vi "xcorr bkp enable.vi"(4 "shift":u8, 5 "Pulse Energy":fxp<+,32,0>=0.99609375, 6 "N":u8, 7 "y":u32, 8 "x":u32, 9 "enable":bool, 10 "lag":u16) -> (1 "Rxy valid":bool, 2 "Rxy":u64, 3 "trigger":bool)   [LabVIEW 2017]
uses:
  <vilib>/rvi/FXPMathLib/basic elements/FxpDiscreteDelay/XNode/nifxpmath_DiscreteDelay.xnode
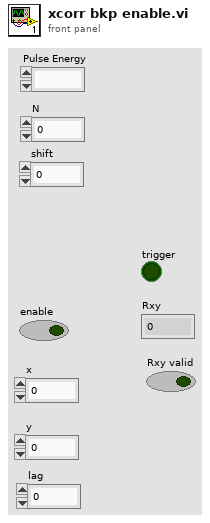
[diagram p1: front panel]
types:
  T1 = cluster{"Q":bool, "Q":bool, "Q":bool, "Q":bool, "Q":bool, "Q":bool, "Q":bool, "Q":bool, "Q":bool, "Q":bool, "Q":bool, "Q":bool, "valid":bool}
  T2 = cluster{"Q":bool, "Q":bool, "Q":bool, "Q":bool, "Q":bool, "Q":bool, "Q":bool, "Q":bool, "Q":bool, "Q":bool, "Q":bool, "Q":bool, "Q":bool}
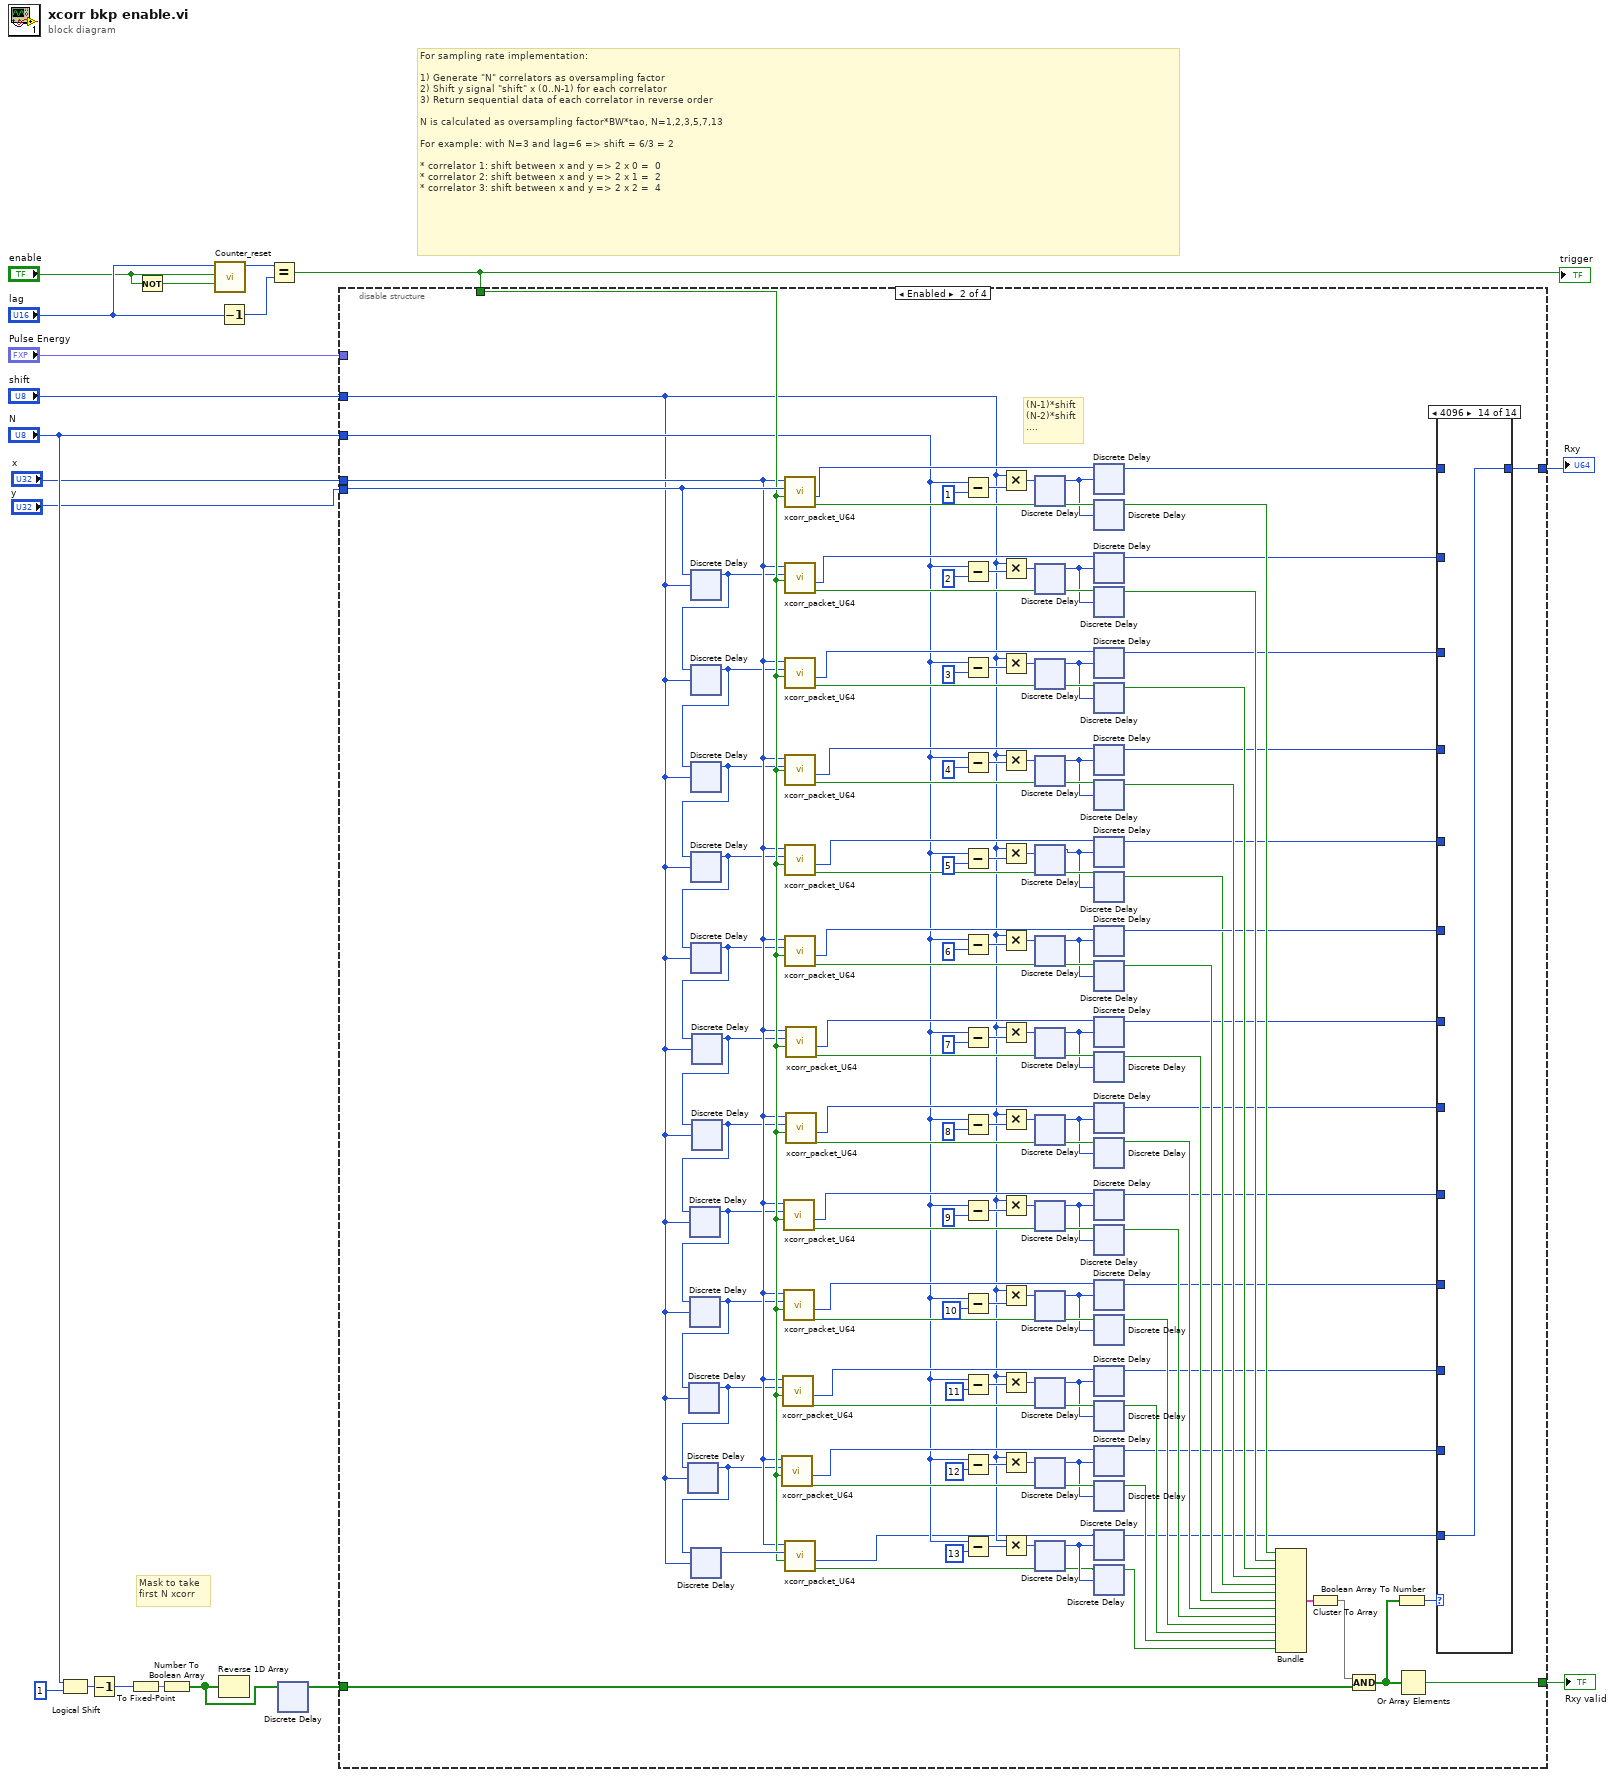
[diagram p0: block diagram]
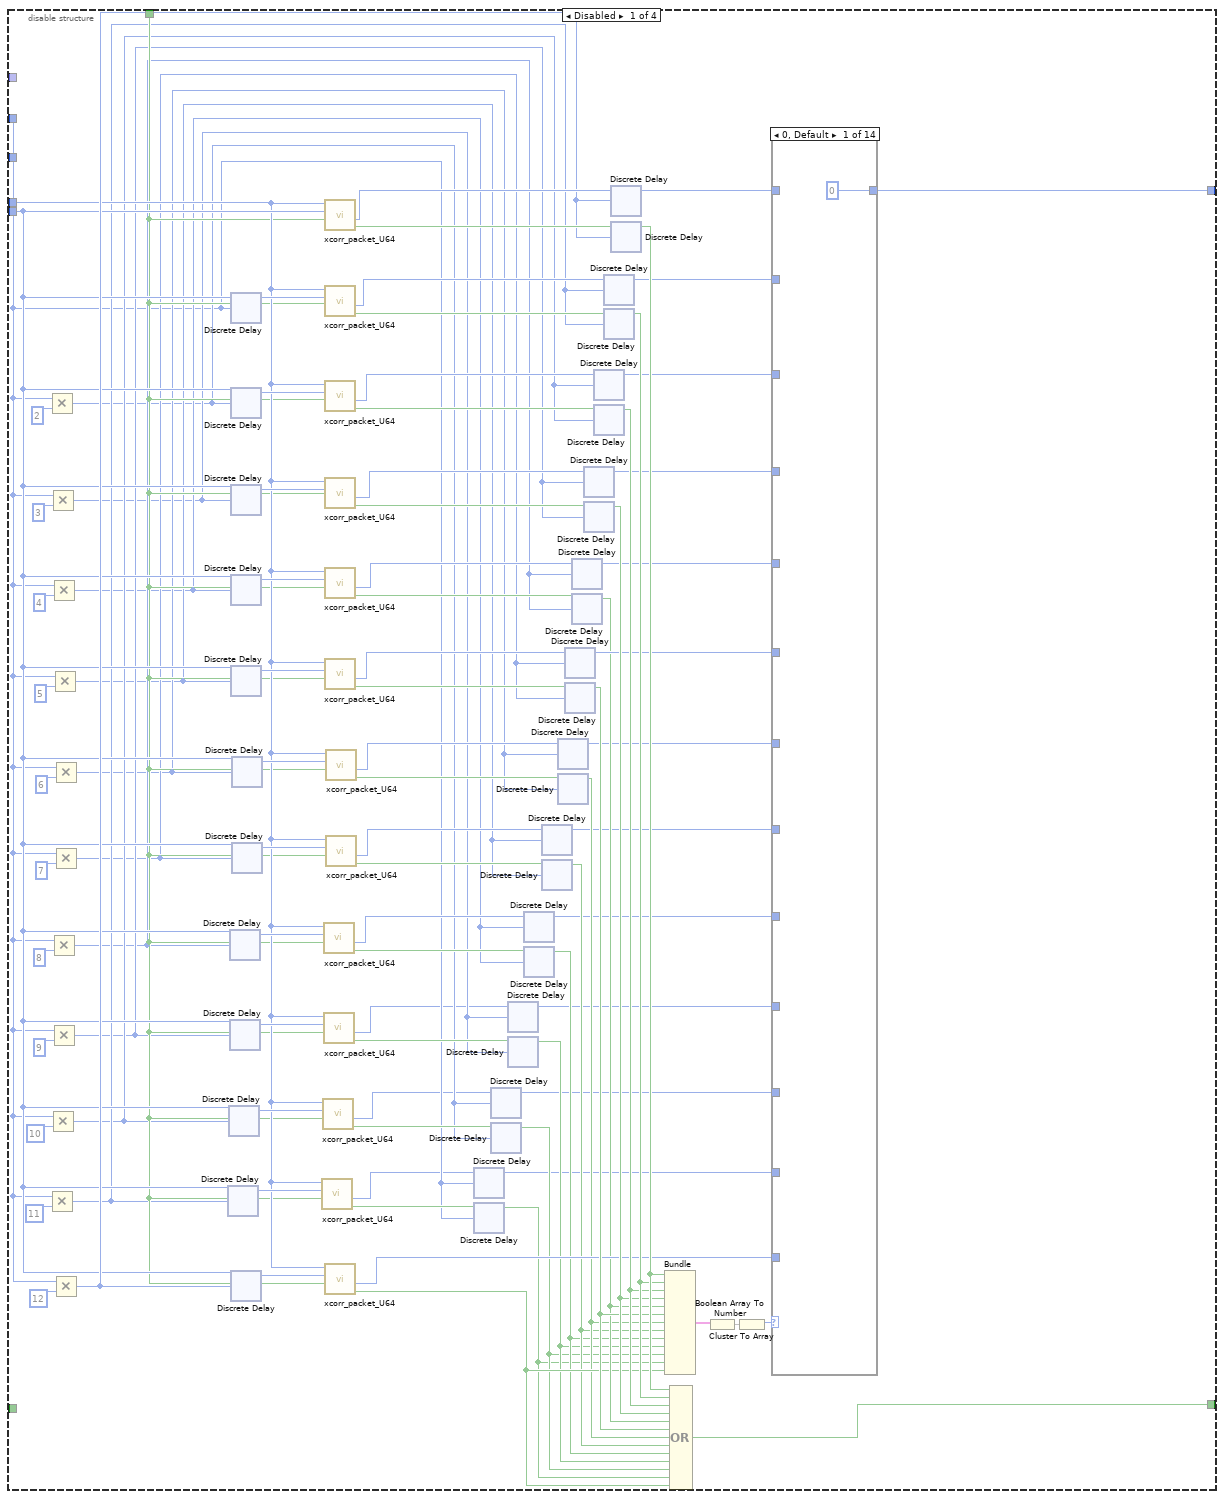
[diagram p2: hidden frame]
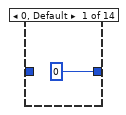
[diagram p16: hidden frame]
diagram:
  # "Mask to take \nfirst N xcorr"
  # "For sampling rate implementation:\n\n1) Generate \"N\" correlators as oversampling factor\n2) Shift y signal \"shift\" x (0..N-1) for each correlator\n3) Return sequential data of each correlator in reverse order\n\nN is calculated as oversampling factor*BW*tao, N=1,2,3,5,7,13\n\nFor example: with N=3 and lag=6 => shift = 6/3 = 2\n\n* correlator 1: shift between x and y => 2 x 0 =  0\n* correlator 2: shift between x and y => 2 x 1 =  2\n* correlator 3: shift between x and y => 2 x 2 =  4"
  n1 = Logical Shift(y="N", x=u16 1) -> (x << y=w8:u16)
  n2 = Decrement(x=w8) -> (x-1=w7:u16)
  n3 = To Fixed-Point(number=w7) -> (fixed-point=w6:fxp<+,13,13>)  [unwired: 1 in]
  n4 = Not(x="enable") -> (.not. x?=w17:bool)
  n5 = Number To Boolean Array(number=w6) -> (Boolean array=w4:bool[])
  n6 = call "Counter_reset.vi"("reset"=w17, "enable"="enable", "limit"="lag") -> ("count"=w18:u16)  [unwired: 8 in]
  n7 = Decrement(x="lag") -> (x-1=w15:u16)
  n8 = Reverse 1D Array(array=w4) -> ()  [unwired: 1 out]
  n9 = Equal?(x=w18, y=w15) -> (x = y?=w12:bool)
  "trigger" <- w12
  n10 = xnode ("Discrete Delay")("D"=w4) -> ("Q"=w10:bool[])
  n11 = disable-structure shown="Enabled" {
    disable-tunnel: [w112 w188 w355 _] -> w19
    disable-tunnel: [w107 w251 w416 _] -> w14
    disable-tunnel: "y" -> [w42 w211 w270 _]
    disable-tunnel: "x" -> [w41 w200 w273 _]
    disable-tunnel: w12 -> [w40 w210 w376 _]
    disable-tunnel: "shift" -> [w28 w131 w298 _]
    disable-tunnel: w10 -> [_ w187 w354 _]
    disable-tunnel: "N" -> [_ w156 w323 _]
    disable-tunnel: "Pulse Energy" -> [_ _ w269 _]
    frame Disabled {
      n12 = Multiply(x=w28, y=u8 2 ("x")) -> (x*y=w29:u8)
      n13 = Multiply(x=w28, y=u8 11 ("x")) -> (x*y=w38:u8)
      n14 = Multiply(x=w28, y=u8 3 ("x")) -> (x*y=w30:u8)
      n15 = Multiply(x=w28, y=u8 10 ("x")) -> (x*y=w37:u8)
      n16 = Multiply(x=w28, y=u8 4 ("x")) -> (x*y=w31:u8)
      n17 = Multiply(x=w28, y=u8 8 ("x")) -> (x*y=w35:u8)
      n18 = Multiply(x=w28, y=u8 9 ("x")) -> (x*y=w36:u8)
      n19 = Multiply(x=w28, y=u8 5 ("x")) -> (x*y=w32:u8)
      n20 = Multiply(x=w28, y=u8 6 ("x")) -> (x*y=w33:u8)
      n21 = Multiply(x=w28, y=u8 7 ("x")) -> (x*y=w34:u8)
      n22 = Multiply(x=w28, y=u8 12 ("x")) -> (x*y=w78:u8)
      n23 = xnode ("Discrete Delay")("D"=w42, "n-1[0..255]"=w38) -> ("Q"=w44:u32)
      n24 = xnode ("Discrete Delay")("D"=w42, "n-1[0..255]"=w37) -> ("Q"=w51:u32)
      n25 = xnode ("Discrete Delay")("D"=w42, "n-1[0..255]"=w35) -> ("Q"=w57:u32)
      n26 = xnode ("Discrete Delay")("D"=w42, "n-1[0..255]"=w36) -> ("Q"=w54:u32)
      n27 = xnode ("Discrete Delay")("D"=w42, "n-1[0..255]"=w28) -> ("Q"=w111:u32)
      n28 = xnode ("Discrete Delay")("D"=w42, "n-1[0..255]"=w29) -> ("Q"=w105:u32)
      n29 = xnode ("Discrete Delay")("D"=w42, "n-1[0..255]"=w30) -> ("Q"=w103:u32)
      n30 = xnode ("Discrete Delay")("D"=w42, "n-1[0..255]"=w31) -> ("Q"=w101:u32)
      n31 = xnode ("Discrete Delay")("D"=w42, "n-1[0..255]"=w32) -> ("Q"=w87:u32)
      n32 = xnode ("Discrete Delay")("D"=w42, "n-1[0..255]"=w78) -> ("Q"=w79:u32)
      n33 = xnode ("Discrete Delay")("D"=w42, "n-1[0..255]"=w33) -> ("Q"=w72:u32)
      n34 = xnode ("Discrete Delay")("D"=w42, "n-1[0..255]"=w34) -> ("Q"=w62:u32)
      n35 = call "xcorr_packet_U64.vi"("x"=w41, "y"=w44, "trigger"=w40) -> ("out"=w20:u64, "valid"=w43:bool)  [unwired: 5 in]
      n36 = call "xcorr_packet_U64.vi"("x"=w41, "y"=w51, "trigger"=w40) -> ("out"=w21:u64, "valid"=w52:bool)  [unwired: 5 in]
      n37 = call "xcorr_packet_U64.vi"("x"=w41, "y"=w57, "trigger"=w40) -> ("out"=w59:u64, "valid"=w58:bool)  [unwired: 5 in]
      n38 = call "xcorr_packet_U64.vi"("x"=w41, "y"=w54, "trigger"=w40) -> ("out"=w22:u64, "valid"=w53:bool)  [unwired: 5 in]
      n39 = call "xcorr_packet_U64.vi"("x"=w41, "y"=w42, "trigger"=w40) -> ("out"=w110:u64, "valid"=w109:bool)  [unwired: 5 in]
      n40 = call "xcorr_packet_U64.vi"("x"=w41, "y"=w111, "trigger"=w40) -> ("out"=w93:u64, "valid"=w98:bool)  [unwired: 5 in]
      n41 = call "xcorr_packet_U64.vi"("x"=w41, "y"=w105, "trigger"=w40) -> ("out"=w92:u64, "valid"=w97:bool)  [unwired: 5 in]
      n42 = call "xcorr_packet_U64.vi"("x"=w41, "y"=w103, "trigger"=w40) -> ("out"=w90:u64, "valid"=w95:bool)  [unwired: 5 in]
      n43 = call "xcorr_packet_U64.vi"("x"=w41, "y"=w101, "trigger"=w40) -> ("out"=w82:u64, "valid"=w76:bool)  [unwired: 5 in]
      n44 = call "xcorr_packet_U64.vi"("x"=w41, "y"=w87, "trigger"=w40) -> ("out"=w84:u64, "valid"=w86:bool)  [unwired: 5 in]
      n45 = call "xcorr_packet_U64.vi"("x"=w41, "y"=w79, "trigger"=w40) -> ("out"=w77:u64, "valid"=w69:bool)  [unwired: 5 in]
      n46 = call "xcorr_packet_U64.vi"("x"=w41, "y"=w72, "trigger"=w40) -> ("out"=w74:u64, "valid"=w73:bool)  [unwired: 5 in]
      n47 = call "xcorr_packet_U64.vi"("x"=w41, "y"=w62, "trigger"=w40) -> ("out"=w60:u64, "valid"=w61:bool)  [unwired: 5 in]
      n48 = xnode ("Discrete Delay")("D"=w20, "n-1[0..255]"=w28) -> ("Q"=w24:u64)
      n49 = xnode ("Discrete Delay")("D"=w43, "n-1[0..255]"=w28) -> ("Q"=w39:bool)
      n50 = xnode ("Discrete Delay")("D"=w21, "n-1[0..255]"=w29) -> ("Q"=w25:u64)
      n51 = xnode ("Discrete Delay")("D"=w52, "n-1[0..255]"=w29) -> ("Q"=w46:bool)
      n52 = xnode ("Discrete Delay")("D"=w22, "n-1[0..255]"=w30) -> ("Q"=w26:u64)
      n53 = xnode ("Discrete Delay")("D"=w53, "n-1[0..255]"=w30) -> ("Q"=w47:bool)
      n54 = xnode ("Discrete Delay")("D"=w59, "n-1[0..255]"=w31) -> ("Q"=w27:u64)
      n55 = xnode ("Discrete Delay")("D"=w58, "n-1[0..255]"=w31) -> ("Q"=w48:bool)
      n56 = xnode ("Discrete Delay")("D"=w60, "n-1[0..255]"=w32) -> ("Q"=w23:u64)
      n57 = xnode ("Discrete Delay")("D"=w61, "n-1[0..255]"=w32) -> ("Q"=w49:bool)
      n58 = xnode ("Discrete Delay")("D"=w74, "n-1[0..255]"=w33) -> ("Q"=w70:u64)
      n59 = xnode ("Discrete Delay")("D"=w73, "n-1[0..255]"=w33) -> ("Q"=w67:bool)
      n60 = xnode ("Discrete Delay")("D"=w84, "n-1[0..255]"=w34) -> ("Q"=w83:u64)
      n61 = xnode ("Discrete Delay")("D"=w86, "n-1[0..255]"=w34) -> ("Q"=w85:bool)
      n62 = xnode ("Discrete Delay")("D"=w82, "n-1[0..255]"=w35) -> ("Q"=w81:u64)
      n63 = xnode ("Discrete Delay")("D"=w76, "n-1[0..255]"=w35) -> ("Q"=w75:bool)
      n64 = xnode ("Discrete Delay")("D"=w90, "n-1[0..255]"=w36) -> ("Q"=w89:u64)
      n65 = xnode ("Discrete Delay")("D"=w95, "n-1[0..255]"=w36) -> ("Q"=w94:bool)
      n66 = xnode ("Discrete Delay")("D"=w92, "n-1[0..255]"=w37) -> ("Q"=w91:u64)
      n67 = xnode ("Discrete Delay")("D"=w97, "n-1[0..255]"=w37) -> ("Q"=w96:bool)
      n68 = xnode ("Discrete Delay")("D"=w93, "n-1[0..255]"=w38) -> ("Q"=w68:u64)
      n69 = xnode ("Discrete Delay")("D"=w98, "n-1[0..255]"=w38) -> ("Q"=w99:bool)
      n70 = xnode ("Discrete Delay")("D"=w110, "n-1[0..255]"=w78) -> ("Q"=w108:u64)
      n71 = xnode ("Discrete Delay")("D"=w109, "n-1[0..255]"=w78) -> ("Q"=w100:bool)
      n72 = Bundle("Q"=w100, "Q"=w99, "Q"=w96, "Q"=w94, "Q"=w75, "Q"=w85, "Q"=w67, "Q"=w49, "Q"=w48, "Q"=w47, "Q"=w46, "Q"=w39, "valid"=w69) -> (w66:T1)  [unwired: 1 in]
      n73 = Compound Arithmetic op=OR(w100, w99, w96, w94, w75, w85, w67, w49, w48, w47, w46, w39, w69) -> (w112:bool)
      n74 = Cluster To Array(cluster=w66) -> (array=w64:bool[])
      n75 = Boolean Array To Number(Boolean array=w64) -> (number=w65:u16)
      n76 = case shown="0, Default" w65 {
        tunnel: [u64 0 ("out") w114 w115 w116 w117 w118 w119 w120 w121 w122 w123 w124 w125 w126] -> w107
        tunnel: w108 -> [_ w114 _ _ _ _ _ _ _ _ _ _ _ _]
        tunnel: w68 -> [_ _ w115 _ _ _ _ _ _ _ _ _ _ _]
        tunnel: w91 -> [_ _ _ w116 _ _ _ _ _ _ _ _ _ _]
        tunnel: w89 -> [_ _ _ _ w117 _ _ _ _ _ _ _ _ _]
        tunnel: w81 -> [_ _ _ _ _ w118 _ _ _ _ _ _ _ _]
        tunnel: w83 -> [_ _ _ _ _ _ w119 _ _ _ _ _ _ _]
        tunnel: w77 -> [_ _ _ _ _ _ _ _ _ _ _ _ _ w126]
        tunnel: w70 -> [_ _ _ _ _ _ _ w120 _ _ _ _ _ _]
        tunnel: w23 -> [_ _ _ _ _ _ _ _ w121 _ _ _ _ _]
        tunnel: w27 -> [_ _ _ _ _ _ _ _ _ w122 _ _ _ _]
        tunnel: w26 -> [_ _ _ _ _ _ _ _ _ _ w123 _ _ _]
        tunnel: w25 -> [_ _ _ _ _ _ _ _ _ _ _ w124 _ _]
        tunnel: w24 -> [_ _ _ _ _ _ _ _ _ _ _ _ w125 _]
        frame 0, Default {
        }
        frame 1 {
        }
        frame 2 {
        }
        frame 4 {
        }
        frame 8 {
        }
        frame 16 {
        }
        frame 32 {
        }
        frame 64 {
        }
        frame 128 {
        }
        frame 256 {
        }
        frame 512 {
        }
        frame 1024 {
        }
        frame 2048 {
        }
        frame 4096 {
        }
      }
    }
    frame Enabled {
      # "(N-1)*shift\n(N-2)*shift\n...."
      n77 = xnode ("Discrete Delay")("D"=w211, "n-1[0..255]"=w131) -> ("Q"=w189:u32)
      n78 = xnode ("Discrete Delay")("D"=w189, "n-1[0..255]"=w131) -> ("Q"=w199:u32)
      n79 = xnode ("Discrete Delay")("D"=w199, "n-1[0..255]"=w131) -> ("Q"=w198:u32)
      n80 = xnode ("Discrete Delay")("D"=w198, "n-1[0..255]"=w131) -> ("Q"=w197:u32)
      n81 = xnode ("Discrete Delay")("D"=w197, "n-1[0..255]"=w131) -> ("Q"=w196:u32)
      n82 = xnode ("Discrete Delay")("D"=w196, "n-1[0..255]"=w131) -> ("Q"=w195:u32)
      n83 = xnode ("Discrete Delay")("D"=w195, "n-1[0..255]"=w131) -> ("Q"=w194:u32)
      n84 = xnode ("Discrete Delay")("D"=w194, "n-1[0..255]"=w131) -> ("Q"=w193:u32)
      n85 = xnode ("Discrete Delay")("D"=w193, "n-1[0..255]"=w131) -> ("Q"=w192:u32)
      n86 = xnode ("Discrete Delay")("D"=w192, "n-1[0..255]"=w131) -> ("Q"=w191:u32)
      n87 = xnode ("Discrete Delay")("D"=w191, "n-1[0..255]"=w131) -> ("Q"=w190:u32)
      n88 = xnode ("Discrete Delay")("D"=w190, "n-1[0..255]"=w131) -> ("Q"=w232:u32)
      n89 = call "xcorr_packet_U64.vi"("x"=w200, "y"=w190, "trigger"=w210) -> ("out"=w201:u64, "valid"=w212:bool)  [unwired: 5 in]
      n90 = call "xcorr_packet_U64.vi"("x"=w200, "y"=w191, "trigger"=w210) -> ("out"=w202:u64, "valid"=w217:bool)  [unwired: 5 in]
      n91 = call "xcorr_packet_U64.vi"("x"=w200, "y"=w193, "trigger"=w210) -> ("out"=w220:u64, "valid"=w219:bool)  [unwired: 5 in]
      n92 = call "xcorr_packet_U64.vi"("x"=w200, "y"=w192, "trigger"=w210) -> ("out"=w203:u64, "valid"=w218:bool)  [unwired: 5 in]
      n93 = call "xcorr_packet_U64.vi"("x"=w200, "y"=w211, "trigger"=w210) -> ("out"=w254:u64, "valid"=w253:bool)  [unwired: 5 in]
      n94 = call "xcorr_packet_U64.vi"("x"=w200, "y"=w189, "trigger"=w210) -> ("out"=w243:u64, "valid"=w248:bool)  [unwired: 5 in]
      n95 = call "xcorr_packet_U64.vi"("x"=w200, "y"=w199, "trigger"=w210) -> ("out"=w242:u64, "valid"=w247:bool)  [unwired: 5 in]
      n96 = call "xcorr_packet_U64.vi"("x"=w200, "y"=w198, "trigger"=w210) -> ("out"=w240:u64, "valid"=w245:bool)  [unwired: 5 in]
      n97 = call "xcorr_packet_U64.vi"("x"=w200, "y"=w197, "trigger"=w210) -> ("out"=w234:u64, "valid"=w231:bool)  [unwired: 5 in]
      n98 = call "xcorr_packet_U64.vi"("x"=w200, "y"=w196, "trigger"=w210) -> ("out"=w236:u64, "valid"=w238:bool)  [unwired: 5 in]
      n99 = call "xcorr_packet_U64.vi"("x"=w200, "y"=w232, "trigger"=w210) -> ("out"=w130:u64, "valid"=w128:bool)  [unwired: 5 in]
      n100 = call "xcorr_packet_U64.vi"("x"=w200, "y"=w195, "trigger"=w210) -> ("out"=w229:u64, "valid"=w228:bool)  [unwired: 5 in]
      n101 = call "xcorr_packet_U64.vi"("x"=w200, "y"=w194, "trigger"=w210) -> ("out"=w221:u64, "valid"=w222:bool)  [unwired: 5 in]
      n102 = Subtract(x=w156, y=u8 1 ("x")) -> (x-y=w183:u8)
      n103 = Subtract(x=w156, y=u8 2 ("x")) -> (x-y=w181:u8)
      n104 = Subtract(x=w156, y=u8 3 ("x")) -> (x-y=w179:u8)
      n105 = Subtract(x=w156, y=u8 4 ("x")) -> (x-y=w177:u8)
      n106 = Subtract(x=w156, y=u8 5 ("x")) -> (x-y=w175:u8)
      n107 = Subtract(x=w156, y=u8 6 ("x")) -> (x-y=w173:u8)
      n108 = Subtract(x=w156, y=u8 7 ("x")) -> (x-y=w171:u8)
      n109 = Subtract(x=w156, y=u8 8 ("x")) -> (x-y=w169:u8)
      n110 = Subtract(x=w156, y=u8 9 ("x")) -> (x-y=w167:u8)
      n111 = Subtract(x=w156, y=u8 10 ("x")) -> (x-y=w165:u8)
      n112 = Subtract(x=w156, y=u8 11 ("x")) -> (x-y=w163:u8)
      n113 = Subtract(x=w156, y=u8 12 ("x")) -> (x-y=w162:u8)
      n114 = Subtract(x=w156, y=u8 13 ("x")) -> (x-y=w157:u8)
      n115 = Multiply(x=w131, y=w183) -> (x*y=w160:u8)
      n116 = Multiply(x=w131, y=w181) -> (x*y=w155:u8)
      n117 = Multiply(x=w131, y=w179) -> (x*y=w153:u8)
      n118 = Multiply(x=w131, y=w177) -> (x*y=w151:u8)
      n119 = Multiply(x=w131, y=w175) -> (x*y=w149:u8)
      n120 = Multiply(x=w131, y=w173) -> (x*y=w147:u8)
      n121 = Multiply(x=w131, y=w171) -> (x*y=w145:u8)
      n122 = Multiply(x=w131, y=w169) -> (x*y=w143:u8)
      n123 = Multiply(x=w131, y=w167) -> (x*y=w141:u8)
      n124 = Multiply(x=w131, y=w165) -> (x*y=w139:u8)
      n125 = Multiply(x=w131, y=w163) -> (x*y=w137:u8)
      n126 = Multiply(x=w131, y=w162) -> (x*y=w135:u8)
      n127 = Multiply(x=w131, y=w157) -> (x*y=w133:u8)
      n128 = xnode ("Discrete Delay")("D"=w160) -> ("Q"=w159:u8)
      n129 = xnode ("Discrete Delay")("D"=w155) -> ("Q"=w154:u8)
      n130 = xnode ("Discrete Delay")("D"=w153) -> ("Q"=w152:u8)
      n131 = xnode ("Discrete Delay")("D"=w151) -> ("Q"=w150:u8)
      n132 = xnode ("Discrete Delay")("D"=w149) -> ("Q"=w148:u8)
      n133 = xnode ("Discrete Delay")("D"=w147) -> ("Q"=w146:u8)
      n134 = xnode ("Discrete Delay")("D"=w145) -> ("Q"=w144:u8)
      n135 = xnode ("Discrete Delay")("D"=w143) -> ("Q"=w142:u8)
      n136 = xnode ("Discrete Delay")("D"=w141) -> ("Q"=w140:u8)
      n137 = xnode ("Discrete Delay")("D"=w139) -> ("Q"=w138:u8)
      n138 = xnode ("Discrete Delay")("D"=w137) -> ("Q"=w136:u8)
      n139 = xnode ("Discrete Delay")("D"=w135) -> ("Q"=w134:u8)
      n140 = xnode ("Discrete Delay")("D"=w133) -> ("Q"=w132:u8)
      n141 = xnode ("Discrete Delay")("D"=w254, "n-1[0..255]"=w159) -> ("Q"=w252:u64)
      n142 = xnode ("Discrete Delay")("D"=w253, "n-1[0..255]"=w159) -> ("Q"=w250:bool)
      n143 = xnode ("Discrete Delay")("D"=w243, "n-1[0..255]"=w154) -> ("Q"=w226:u64)
      n144 = xnode ("Discrete Delay")("D"=w248, "n-1[0..255]"=w154) -> ("Q"=w249:bool)
      n145 = xnode ("Discrete Delay")("D"=w242, "n-1[0..255]"=w152) -> ("Q"=w241:u64)
      n146 = xnode ("Discrete Delay")("D"=w247, "n-1[0..255]"=w152) -> ("Q"=w246:bool)
      n147 = xnode ("Discrete Delay")("D"=w240, "n-1[0..255]"=w150) -> ("Q"=w239:u64)
      n148 = xnode ("Discrete Delay")("D"=w245, "n-1[0..255]"=w150) -> ("Q"=w244:bool)
      n149 = xnode ("Discrete Delay")("D"=w234, "n-1[0..255]"=w148) -> ("Q"=w233:u64)
      n150 = xnode ("Discrete Delay")("D"=w231, "n-1[0..255]"=w148) -> ("Q"=w230:bool)
      n151 = xnode ("Discrete Delay")("D"=w236, "n-1[0..255]"=w146) -> ("Q"=w235:u64)
      n152 = xnode ("Discrete Delay")("D"=w238, "n-1[0..255]"=w146) -> ("Q"=w237:bool)
      n153 = xnode ("Discrete Delay")("D"=w229, "n-1[0..255]"=w144) -> ("Q"=w227:u64)
      n154 = xnode ("Discrete Delay")("D"=w228, "n-1[0..255]"=w144) -> ("Q"=w225:bool)
      n155 = xnode ("Discrete Delay")("D"=w221, "n-1[0..255]"=w142) -> ("Q"=w204:u64)
      n156 = xnode ("Discrete Delay")("D"=w222, "n-1[0..255]"=w142) -> ("Q"=w216:bool)
      n157 = xnode ("Discrete Delay")("D"=w220, "n-1[0..255]"=w140) -> ("Q"=w208:u64)
      n158 = xnode ("Discrete Delay")("D"=w219, "n-1[0..255]"=w140) -> ("Q"=w215:bool)
      n159 = xnode ("Discrete Delay")("D"=w203, "n-1[0..255]"=w138) -> ("Q"=w207:u64)
      n160 = xnode ("Discrete Delay")("D"=w218, "n-1[0..255]"=w138) -> ("Q"=w214:bool)
      n161 = xnode ("Discrete Delay")("D"=w202, "n-1[0..255]"=w136) -> ("Q"=w206:u64)
      n162 = xnode ("Discrete Delay")("D"=w217, "n-1[0..255]"=w136) -> ("Q"=w213:bool)
      n163 = xnode ("Discrete Delay")("D"=w201, "n-1[0..255]"=w134) -> ("Q"=w205:u64)
      n164 = xnode ("Discrete Delay")("D"=w212, "n-1[0..255]"=w134) -> ("Q"=w209:bool)
      n165 = xnode ("Discrete Delay")("D"=w130, "n-1[0..255]"=w132) -> ("Q"=w129:u64)
      n166 = xnode ("Discrete Delay")("D"=w128, "n-1[0..255]"=w132) -> ("Q"=w127:bool)
      n167 = Bundle("Q"=w250, "Q"=w249, "Q"=w246, "Q"=w244, "Q"=w230, "Q"=w237, "Q"=w225, "Q"=w216, "Q"=w215, "Q"=w214, "Q"=w213, "Q"=w209, "Q"=w127) -> (w224:T2)  [unwired: 1 in]
      n168 = Cluster To Array(cluster=w224) -> (array=w186:bool[])
      n169 = Compound Arithmetic op=AND(w186, w187) -> (w185:bool[])
      n170 = Boolean Array To Number(Boolean array=w185) -> (number=w223:u16)
      n171 = Or Array Elements(Boolean array=w185) -> (logical OR=w188:bool)
      n172 = case shown="4096" w223 {
        tunnel: [u64 0 ("out") w256 w257 w258 w259 w260 w261 w262 w263 w264 w265 w266 w267 w268] -> w251
        tunnel: w252 -> [_ w256 _ _ _ _ _ _ _ _ _ _ _ _]
        tunnel: w226 -> [_ _ w257 _ _ _ _ _ _ _ _ _ _ _]
        tunnel: w241 -> [_ _ _ w258 _ _ _ _ _ _ _ _ _ _]
        tunnel: w239 -> [_ _ _ _ w259 _ _ _ _ _ _ _ _ _]
        tunnel: w233 -> [_ _ _ _ _ w260 _ _ _ _ _ _ _ _]
        tunnel: w235 -> [_ _ _ _ _ _ w261 _ _ _ _ _ _ _]
        tunnel: w129 -> [_ _ _ _ _ _ _ _ _ _ _ _ _ w268]
        tunnel: w227 -> [_ _ _ _ _ _ _ w262 _ _ _ _ _ _]
        tunnel: w204 -> [_ _ _ _ _ _ _ _ w263 _ _ _ _ _]
        tunnel: w208 -> [_ _ _ _ _ _ _ _ _ w264 _ _ _ _]
        tunnel: w207 -> [_ _ _ _ _ _ _ _ _ _ w265 _ _ _]
        tunnel: w206 -> [_ _ _ _ _ _ _ _ _ _ _ w266 _ _]
        tunnel: w205 -> [_ _ _ _ _ _ _ _ _ _ _ _ w267 _]
        frame 0, Default {
        }
        frame 1 {
        }
        frame 2 {
        }
        frame 4 {
        }
        frame 8 {
        }
        frame 16 {
        }
        frame 32 {
        }
        frame 64 {
        }
        frame 128 {
        }
        frame 256 {
        }
        frame 512 {
        }
        frame 1024 {
        }
        frame 2048 {
        }
        frame 4096 {
        }
      }
    }
    frame Disabled {
      # "(N-1)*shift\n(N-2)*shift\n...."
      n173 = Split Number(x=w273) -> (hi(x)=w290:u16, lo(x)=w291:u16)
      n174 = Split Number(x=w270) -> (hi(x)=w292:u16, lo(x)=w293:u16)
      n175 = To Word Integer(number=w290) -> (16bit integer=w276:i16)
      n176 = To Word Integer(number=w291) -> (16bit integer=w277:i16)
      n177 = To Word Integer(number=w292) -> (16bit integer=w275:i16)
      n178 = To Word Integer(number=w293) -> (16bit integer=w274:i16)
      n179 = Integer to Fixed-Point Cast(integer=w276) -> (fixed-point=w289:fxp<+/-,16,16>)  [unwired: 1 in]
      n180 = Integer to Fixed-Point Cast(integer=w277) -> (fixed-point=w288:fxp<+/-,16,16>)  [unwired: 1 in]
      n181 = Integer to Fixed-Point Cast(integer=w275) -> (fixed-point=w286:fxp<+/-,16,16>)  [unwired: 1 in]
      n182 = Integer to Fixed-Point Cast(integer=w274) -> (fixed-point=w287:fxp<+/-,16,16>)  [unwired: 1 in]
      n183 = Multiply(x=w269, y=w289) -> (x*y=w285:fxp<+/-,16,1>)
      n184 = Multiply(x=w269, y=w288) -> (x*y=w283:fxp<+/-,16,1>)
      n185 = Multiply(x=w269, y=w286) -> (x*y=w281:fxp<+/-,16,1>)
      n186 = Multiply(x=w269, y=w287) -> (x*y=w278:fxp<+/-,16,1>)
      n187 = Fixed-Point to Integer Cast(1:w285) -> (0:w284:i16)
      n188 = Fixed-Point to Integer Cast(1:w283) -> (0:w282:i16)
      n189 = Fixed-Point to Integer Cast(1:w281) -> (0:w280:i16)
      n190 = Fixed-Point to Integer Cast(1:w278) -> (0:w279:i16)
      n191 = Join Numbers(hi=w284, lo=w282) -> ((hi.lo)=w272:u32)
      n192 = Join Numbers(hi=w280, lo=w279) -> ((hi.lo)=w271:u32)
      n193 = xnode ("Discrete Delay")("D"=w271, "n-1[0..255]"=w298) -> ("Q"=w356:u32)
      n194 = xnode ("Discrete Delay")("D"=w356, "n-1[0..255]"=w298) -> ("Q"=w366:u32)
      n195 = xnode ("Discrete Delay")("D"=w366, "n-1[0..255]"=w298) -> ("Q"=w365:u32)
      n196 = xnode ("Discrete Delay")("D"=w365, "n-1[0..255]"=w298) -> ("Q"=w364:u32)
      n197 = xnode ("Discrete Delay")("D"=w364, "n-1[0..255]"=w298) -> ("Q"=w363:u32)
      n198 = xnode ("Discrete Delay")("D"=w363, "n-1[0..255]"=w298) -> ("Q"=w362:u32)
      n199 = xnode ("Discrete Delay")("D"=w362, "n-1[0..255]"=w298) -> ("Q"=w361:u32)
      n200 = xnode ("Discrete Delay")("D"=w361, "n-1[0..255]"=w298) -> ("Q"=w360:u32)
      n201 = xnode ("Discrete Delay")("D"=w360, "n-1[0..255]"=w298) -> ("Q"=w359:u32)
      n202 = xnode ("Discrete Delay")("D"=w359, "n-1[0..255]"=w298) -> ("Q"=w358:u32)
      n203 = xnode ("Discrete Delay")("D"=w358, "n-1[0..255]"=w298) -> ("Q"=w357:u32)
      n204 = xnode ("Discrete Delay")("D"=w357, "n-1[0..255]"=w298) -> ("Q"=w397:u32)
      n205 = call "xcorr_packet_FXP.vi"("x"=w272, "y"=w357, "trigger"=w376) -> ("out"=w367:u64, "valid"=w377:bool)  [unwired: 5 in]
      n206 = call "xcorr_packet_FXP.vi"("x"=w272, "y"=w358, "trigger"=w376) -> ("out"=w368:u64, "valid"=w382:bool)  [unwired: 5 in]
      n207 = call "xcorr_packet_FXP.vi"("x"=w272, "y"=w360, "trigger"=w376) -> ("out"=w385:u64, "valid"=w384:bool)  [unwired: 5 in]
      n208 = call "xcorr_packet_FXP.vi"("x"=w272, "y"=w359, "trigger"=w376) -> ("out"=w369:u64, "valid"=w383:bool)  [unwired: 5 in]
      n209 = call "xcorr_packet_FXP.vi"("x"=w272, "y"=w271, "trigger"=w376) -> ("out"=w419:u64, "valid"=w418:bool)  [unwired: 5 in]
      n210 = call "xcorr_packet_FXP.vi"("x"=w272, "y"=w356, "trigger"=w376) -> ("out"=w408:u64, "valid"=w413:bool)  [unwired: 5 in]
      n211 = call "xcorr_packet_FXP.vi"("x"=w272, "y"=w366, "trigger"=w376) -> ("out"=w407:u64, "valid"=w412:bool)  [unwired: 5 in]
      n212 = call "xcorr_packet_FXP.vi"("x"=w272, "y"=w365, "trigger"=w376) -> ("out"=w405:u64, "valid"=w410:bool)  [unwired: 5 in]
      n213 = call "xcorr_packet_FXP.vi"("x"=w272, "y"=w364, "trigger"=w376) -> ("out"=w399:u64, "valid"=w396:bool)  [unwired: 5 in]
      n214 = call "xcorr_packet_FXP.vi"("x"=w272, "y"=w363, "trigger"=w376) -> ("out"=w401:u64, "valid"=w403:bool)  [unwired: 5 in]
      n215 = call "xcorr_packet_FXP.vi"("x"=w272, "y"=w397, "trigger"=w376) -> ("out"=w297:u64, "valid"=w295:bool)  [unwired: 5 in]
      n216 = call "xcorr_packet_FXP.vi"("x"=w272, "y"=w362, "trigger"=w376) -> ("out"=w394:u64, "valid"=w393:bool)  [unwired: 5 in]
      n217 = call "xcorr_packet_FXP.vi"("x"=w272, "y"=w361, "trigger"=w376) -> ("out"=w386:u64, "valid"=w387:bool)  [unwired: 5 in]
      n218 = Subtract(x=w323, y=u8 1 ("x")) -> (x-y=w350:u8)
      n219 = Subtract(x=w323, y=u8 2 ("x")) -> (x-y=w348:u8)
      n220 = Subtract(x=w323, y=u8 3 ("x")) -> (x-y=w346:u8)
      n221 = Subtract(x=w323, y=u8 4 ("x")) -> (x-y=w344:u8)
      n222 = Subtract(x=w323, y=u8 5 ("x")) -> (x-y=w342:u8)
      n223 = Subtract(x=w323, y=u8 6 ("x")) -> (x-y=w340:u8)
      n224 = Subtract(x=w323, y=u8 7 ("x")) -> (x-y=w338:u8)
      n225 = Subtract(x=w323, y=u8 8 ("x")) -> (x-y=w336:u8)
      n226 = Subtract(x=w323, y=u8 9 ("x")) -> (x-y=w334:u8)
      n227 = Subtract(x=w323, y=u8 10 ("x")) -> (x-y=w332:u8)
      n228 = Subtract(x=w323, y=u8 11 ("x")) -> (x-y=w330:u8)
      n229 = Subtract(x=w323, y=u8 12 ("x")) -> (x-y=w329:u8)
      n230 = Subtract(x=w323, y=u8 13 ("x")) -> (x-y=w324:u8)
      n231 = Multiply(x=w298, y=w350) -> (x*y=w327:u8)
      n232 = Multiply(x=w298, y=w348) -> (x*y=w322:u8)
      n233 = Multiply(x=w298, y=w346) -> (x*y=w320:u8)
      n234 = Multiply(x=w298, y=w344) -> (x*y=w318:u8)
      n235 = Multiply(x=w298, y=w342) -> (x*y=w316:u8)
      n236 = Multiply(x=w298, y=w340) -> (x*y=w314:u8)
      n237 = Multiply(x=w298, y=w338) -> (x*y=w312:u8)
      n238 = Multiply(x=w298, y=w336) -> (x*y=w310:u8)
      n239 = Multiply(x=w298, y=w334) -> (x*y=w308:u8)
      n240 = Multiply(x=w298, y=w332) -> (x*y=w306:u8)
      n241 = Multiply(x=w298, y=w330) -> (x*y=w304:u8)
      n242 = Multiply(x=w298, y=w329) -> (x*y=w302:u8)
      n243 = Multiply(x=w298, y=w324) -> (x*y=w300:u8)
      n244 = xnode ("Discrete Delay")("D"=w327) -> ("Q"=w326:u8)
      n245 = xnode ("Discrete Delay")("D"=w322) -> ("Q"=w321:u8)
      n246 = xnode ("Discrete Delay")("D"=w320) -> ("Q"=w319:u8)
      n247 = xnode ("Discrete Delay")("D"=w318) -> ("Q"=w317:u8)
      n248 = xnode ("Discrete Delay")("D"=w316) -> ("Q"=w315:u8)
      n249 = xnode ("Discrete Delay")("D"=w314) -> ("Q"=w313:u8)
      n250 = xnode ("Discrete Delay")("D"=w312) -> ("Q"=w311:u8)
      n251 = xnode ("Discrete Delay")("D"=w310) -> ("Q"=w309:u8)
      n252 = xnode ("Discrete Delay")("D"=w308) -> ("Q"=w307:u8)
      n253 = xnode ("Discrete Delay")("D"=w306) -> ("Q"=w305:u8)
      n254 = xnode ("Discrete Delay")("D"=w304) -> ("Q"=w303:u8)
      n255 = xnode ("Discrete Delay")("D"=w302) -> ("Q"=w301:u8)
      n256 = xnode ("Discrete Delay")("D"=w300) -> ("Q"=w299:u8)
      n257 = xnode ("Discrete Delay")("D"=w419, "n-1[0..255]"=w326) -> ("Q"=w417:u64)
      n258 = xnode ("Discrete Delay")("D"=w418, "n-1[0..255]"=w326) -> ("Q"=w415:bool)
      n259 = xnode ("Discrete Delay")("D"=w408, "n-1[0..255]"=w321) -> ("Q"=w391:u64)
      n260 = xnode ("Discrete Delay")("D"=w413, "n-1[0..255]"=w321) -> ("Q"=w414:bool)
      n261 = xnode ("Discrete Delay")("D"=w407, "n-1[0..255]"=w319) -> ("Q"=w406:u64)
      n262 = xnode ("Discrete Delay")("D"=w412, "n-1[0..255]"=w319) -> ("Q"=w411:bool)
      n263 = xnode ("Discrete Delay")("D"=w405, "n-1[0..255]"=w317) -> ("Q"=w404:u64)
      n264 = xnode ("Discrete Delay")("D"=w410, "n-1[0..255]"=w317) -> ("Q"=w409:bool)
      n265 = xnode ("Discrete Delay")("D"=w399, "n-1[0..255]"=w315) -> ("Q"=w398:u64)
      n266 = xnode ("Discrete Delay")("D"=w396, "n-1[0..255]"=w315) -> ("Q"=w395:bool)
      n267 = xnode ("Discrete Delay")("D"=w401, "n-1[0..255]"=w313) -> ("Q"=w400:u64)
      n268 = xnode ("Discrete Delay")("D"=w403, "n-1[0..255]"=w313) -> ("Q"=w402:bool)
      n269 = xnode ("Discrete Delay")("D"=w394, "n-1[0..255]"=w311) -> ("Q"=w392:u64)
      n270 = xnode ("Discrete Delay")("D"=w393, "n-1[0..255]"=w311) -> ("Q"=w390:bool)
      n271 = xnode ("Discrete Delay")("D"=w386, "n-1[0..255]"=w309) -> ("Q"=w370:u64)
      n272 = xnode ("Discrete Delay")("D"=w387, "n-1[0..255]"=w309) -> ("Q"=w381:bool)
      n273 = xnode ("Discrete Delay")("D"=w385, "n-1[0..255]"=w307) -> ("Q"=w374:u64)
      n274 = xnode ("Discrete Delay")("D"=w384, "n-1[0..255]"=w307) -> ("Q"=w380:bool)
      n275 = xnode ("Discrete Delay")("D"=w369, "n-1[0..255]"=w305) -> ("Q"=w373:u64)
      n276 = xnode ("Discrete Delay")("D"=w383, "n-1[0..255]"=w305) -> ("Q"=w379:bool)
      n277 = xnode ("Discrete Delay")("D"=w368, "n-1[0..255]"=w303) -> ("Q"=w372:u64)
      n278 = xnode ("Discrete Delay")("D"=w382, "n-1[0..255]"=w303) -> ("Q"=w378:bool)
      n279 = xnode ("Discrete Delay")("D"=w367, "n-1[0..255]"=w301) -> ("Q"=w371:u64)
      n280 = xnode ("Discrete Delay")("D"=w377, "n-1[0..255]"=w301) -> ("Q"=w375:bool)
      n281 = xnode ("Discrete Delay")("D"=w297, "n-1[0..255]"=w299) -> ("Q"=w296:u64)
      n282 = xnode ("Discrete Delay")("D"=w295, "n-1[0..255]"=w299) -> ("Q"=w294:bool)
      n283 = Bundle("Q"=w415, "Q"=w414, "Q"=w411, "Q"=w409, "Q"=w395, "Q"=w402, "Q"=w390, "Q"=w381, "Q"=w380, "Q"=w379, "Q"=w378, "Q"=w375, "Q"=w294) -> (w389:T2)  [unwired: 1 in]
      n284 = Cluster To Array(cluster=w389) -> (array=w353:bool[])
      n285 = Compound Arithmetic op=AND(w353, w354) -> (w352:bool[])
      n286 = Boolean Array To Number(Boolean array=w352) -> (number=w388:u16)
      n287 = Or Array Elements(Boolean array=w352) -> (logical OR=w355:bool)
      n288 = case shown="4096" w388 {
        tunnel: [u64 0 ("out") w421 w422 w423 w424 w425 w426 w427 w428 w429 w430 w431 w432 w433] -> w416
        tunnel: w417 -> [_ w421 _ _ _ _ _ _ _ _ _ _ _ _]
        tunnel: w391 -> [_ _ w422 _ _ _ _ _ _ _ _ _ _ _]
        tunnel: w406 -> [_ _ _ w423 _ _ _ _ _ _ _ _ _ _]
        tunnel: w404 -> [_ _ _ _ w424 _ _ _ _ _ _ _ _ _]
        tunnel: w398 -> [_ _ _ _ _ w425 _ _ _ _ _ _ _ _]
        tunnel: w400 -> [_ _ _ _ _ _ w426 _ _ _ _ _ _ _]
        tunnel: w296 -> [_ _ _ _ _ _ _ _ _ _ _ _ _ w433]
        tunnel: w392 -> [_ _ _ _ _ _ _ w427 _ _ _ _ _ _]
        tunnel: w370 -> [_ _ _ _ _ _ _ _ w428 _ _ _ _ _]
        tunnel: w374 -> [_ _ _ _ _ _ _ _ _ w429 _ _ _ _]
        tunnel: w373 -> [_ _ _ _ _ _ _ _ _ _ w430 _ _ _]
        tunnel: w372 -> [_ _ _ _ _ _ _ _ _ _ _ w431 _ _]
        tunnel: w371 -> [_ _ _ _ _ _ _ _ _ _ _ _ w432 _]
        frame 0, Default {
        }
        frame 1 {
        }
        frame 2 {
        }
        frame 4 {
        }
        frame 8 {
        }
        frame 16 {
        }
        frame 32 {
        }
        frame 64 {
        }
        frame 128 {
        }
        frame 256 {
        }
        frame 512 {
        }
        frame 1024 {
        }
        frame 2048 {
        }
        frame 4096 {
        }
      }
    }
    frame Disabled {
    }
  }
  "Rxy valid" <- w19
  "Rxy" <- w14
